vi "Engine Out - HPCR.vi"(4 "Control Inputs":T2={"Engine Speed [RPM]"=0.0, "Engine Status"=enum."STALLED", "Load Control \nMode"=enum."Max Speed Governor", "dt(s)"=0.0, "Number of Cylinders"=0, "Engine Displacement [cc]"=0.0, "StoichAFR"=0.0, "Q.LHV Fuel [kJ/kg]"=0.0, "BattV PSU [V]"=0.0, "12V PSU [V]"=0.0, "5V PSU [V]"=0.0, "Pedal Position [%]"=0.0, "Oil Pressure [kPa]"=0.0, "Oil Temp [C]"=0.0, "Oil Level [%]"=0.0, "Engine Coolant Temp (ECT) [C]"=0.0, "Engine Coolant Pressure [kPa]"=0.0, "Rail Pressure [bar]"=0.0, "Fuel Pressure [kPa]"=0.0, "Fuel Temp [C]"=0.0, "Vacuum Pressure [kPa]"=0.0, "Throttle Position [%]"=0.0, "Cam1 Advance [CAD]"=0.0, "Cam2 Advance [CAD]"=0.0, "Cam3 Advance [CAD]"=0.0, "Cam4 Advance [CAD]"=0.0, "CA50 Control Output [CAD]"=[], "CA50 Control Output Valid"=[], "Intake Air Temp (IAT) [C]"=0.0, "Barometric Air Pressure [kPa]"=0.0, "Intake Air Rel. Humidity [%]"=0.0, "Mass Air Flow (MAF) [kg/hr]"=0.0, "Turbo Inlet Air Pressure [kPa]"=0.0, "Turbo Inlet Air Temp [C]"=0.0, "Turbo Outlet Air Pressure [kPa]"=0.0, "Turbo Outlet Air Temp [C]"=0.0, "CAC Outlet Pressure [kPa]"=0.0, "CAC Outlet Temp [C]"=0.0, "Intake Manifold Pressure (MAP) [kPa]"=0.0, "Intake Manifold Temp (MAT) [C]"=0.0, "Exhaust Manifold Pressure [kPa]"=0.0, "Exhaust Manifold Temp [C]"=0.0, "HighP EGR Cooler Outlet Pressure [kPa]"=0.0, "HighP EGR Cooler Outlet Temp [C]"=0.0, "HighP EGR Differential Pressure [kPa]"=0.0, "HighP EGR Valve Position [%]"=0.0, "Turbo Outlet Exhaust Pressure [kPa]"=0.0, "Turbo Outlet Exhaust Temp [C]"=0.0, "VGT Position 1 [%]"=0.0, "VGT Position 2 [%]"=0.0, "Turbo Speed 1 [RPM]"=0.0, "Turbo Speed 2 [RPM]"=0.0, "LowP EGR Differential Pressure [kPa]"=0.0, "LowP EGR Valve Position [%]"=0.0, "UEGO1Lambda"=0.0, "UEGO1_Hot"=FALSE, "UEGO2Lambda"=0.0, "UEGO2_Hot"=FALSE, "Knock Intensity"=[], "Knock"=[]} {"Knock Intensity" format="%.2f"; "CA50 Control Output [CAD]" format="%.2f"; "Exhaust Manifold Temp [C]" format="%#_6f"; "UEGO2Lambda" format="%.2f"; "Intake Manifold Temp (MAT) [C]" format="%#_6f"; "UEGO1Lambda" format="%.2f"}, 7 "Rail Pressure Setpoint [bar]":sgl format="%.2f") -> (2 "HPV LS Output":T1, 3 "IMV LS Output":T1)   [LabVIEW 2015, in "ECS-RT.lvlib"]
uses:
  ECS-RT.lvlib
  Typedefs/Control Inputs/Control Inputs.ctl
  Typedefs/EPT/Engine Status.ctl
  Typedefs/MISC/Load Control Mode.ctl
  Typedefs/Raw Outputs/LS.ctl
  ECS-Shared.lvlib
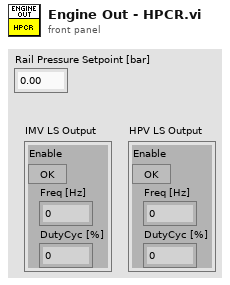
[diagram p1: front panel]
types:
  T1 = typedef "ECS-Shared.lvlib/LS.ctl" = cluster{"Enable":bool, "Freq [Hz]":sgl, "DutyCyc [%]":sgl}
  T2 = typedef "ECS-Shared.lvlib/Control Inputs.ctl" = cluster{"Engine Speed [RPM]":sgl, "Engine Status":T3, "Load Control \nMode":T4, "dt(s)":sgl, "Number of Cylinders":u8, "Engine Displacement [cc]":sgl, "StoichAFR":sgl, "Q.LHV Fuel [kJ/kg]":sgl, "BattV PSU [V]":sgl, "12V PSU [V]":sgl, "5V PSU [V]":sgl, "Pedal Position [%]":sgl, "Oil Pressure [kPa]":sgl, "Oil Temp [C]":sgl, "Oil Level [%]":sgl, "Engine Coolant Temp (ECT) [C]":sgl, "Engine Coolant Pressure [kPa]":sgl, "Rail Pressure [bar]":sgl, "Fuel Pressure [kPa]":sgl, "Fuel Temp [C]":sgl, "Vacuum Pressure [kPa]":sgl, "Throttle Position [%]":sgl, "Cam1 Advance [CAD]":sgl, "Cam2 Advance [CAD]":sgl, "Cam3 Advance [CAD]":sgl, "Cam4 Advance [CAD]":sgl, "CA50 Control Output [CAD]":sgl[], "CA50 Control Output Valid":bool[], "Intake Air Temp (IAT) [C]":sgl, "Barometric Air Pressure [kPa]":sgl, "Intake Air Rel. Humidity [%]":sgl, "Mass Air Flow (MAF) [kg/hr]":sgl, "Turbo Inlet Air Pressure [kPa]":sgl, "Turbo Inlet Air Temp [C]":sgl, "Turbo Outlet Air Pressure [kPa]":sgl, "Turbo Outlet Air Temp [C]":sgl, "CAC Outlet Pressure [kPa]":sgl, "CAC Outlet Temp [C]":sgl, "Intake Manifold Pressure (MAP) [kPa]":sgl, "Intake Manifold Temp (MAT) [C]":sgl, "Exhaust Manifold Pressure [kPa]":sgl, "Exhaust Manifold Temp [C]":sgl, "HighP EGR Cooler Outlet Pressure [kPa]":sgl, "HighP EGR Cooler Outlet Temp [C]":sgl, "HighP EGR Differential Pressure [kPa]":sgl, "HighP EGR Valve Position [%]":sgl, "Turbo Outlet Exhaust Pressure [kPa]":sgl, "Turbo Outlet Exhaust Temp [C]":sgl, "VGT Position 1 [%]":sgl, "VGT Position 2 [%]":sgl, "Turbo Speed 1 [RPM]":sgl, "Turbo Speed 2 [RPM]":sgl, "LowP EGR Differential Pressure [kPa]":sgl, "LowP EGR Valve Position [%]":sgl, "UEGO1Lambda":sgl, "UEGO1_Hot":bool, "UEGO2Lambda":sgl, "UEGO2_Hot":bool, "Knock Intensity":sgl[], "Knock":bool[]}
  T3 = typedef "ECS-Shared.lvlib/Engine Status.ctl" = enum16{"OFF", "STALLED", "CRANKING", "RUNNING", "ACCEL", "DECEL", "SAFE"}
  T4 = typedef "ECS-Shared.lvlib/Load Control Mode.ctl" = enum16{"No Governor", "Min Speed Governor", "Max Speed Governor"}
  T5 = cluster{"PID_Kp":sgl, "PID_Ti":sgl, "PID_Td":sgl, "PID_FF":sgl, "Non-PID_FF":sgl, "PID_Min":sgl, "PID_Max":sgl}
  T6 = cluster{"BattV [V]":sgl, "ValveNominalResitance":sgl, "Min Duty Cycle":sgl, "Manual Max Duty Cycle":sgl, "Manual Duty Cycle":sgl, "Duty Cycle Override":bool, "Drive Frequency":sgl}
  T7 = cluster{"DutyCycle_Output":sgl, "Calculated Max Duty Cycle":sgl, "Valve Current Flow":sgl, "PID_Output":sgl}
  T8 = cluster{"ProportionalAction":sgl, "IntegralAction":sgl, "DerivativeAction":sgl}
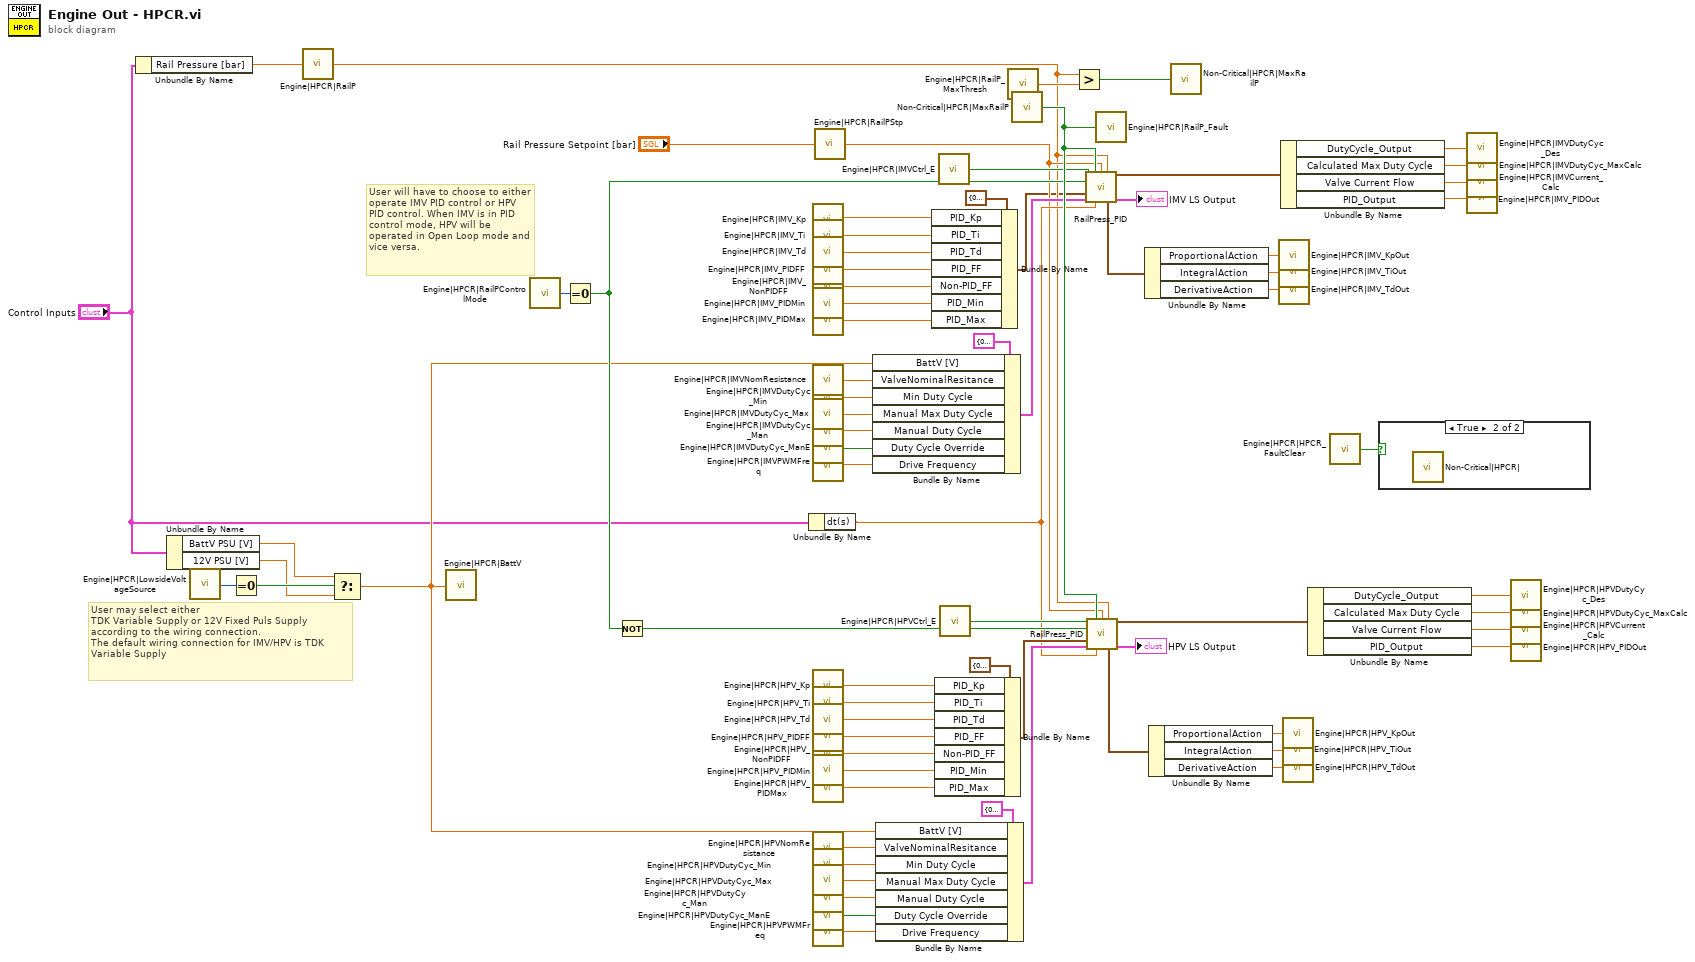
[diagram p0: block diagram]
diagram:
  # "User will have to choose to either operate IMV PID control or HPV PID control. When IMV is in PID control mode, HPV will be operated in Open Loop mode and vice versa."
  # "User may select either\nTDK Variable Supply or 12V Fixed Puls Supply\naccording to the wiring connection.\nThe default wiring connection for IMV/HPV is TDK Variable Supply"
  n1 = Unbundle By Name("Control Inputs") -> ("Rail Pressure [bar]"=w4:sgl)
  n2 = Unbundle By Name("Control Inputs") -> ("BattV PSU [V]"=w11:sgl, "12V PSU [V]"=w10:sgl)
  n3 = call "Engine|HPCR|LowsideVoltageSource"() -> ("Value"=w14:u32)
  n4 = Equal To 0?(x=w14) -> (x = 0?=w13:bool)
  n5 = call "Engine|HPCR|RailP"("Value"=w4) -> ()
  n6 = Select(t=w11, s=w13, f=w10) -> (s? t:f=w12:sgl)
  n7 = call "Engine|HPCR|BattV"("Value"=w12) -> ()
  n8 = call "Engine|HPCR|RailPControlMode"() -> ("Value"=w58:u32)
  n9 = Equal To 0?(x=w58) -> (x = 0?=w59:bool)
  n10 = Not(x=w59) -> (.not. x?=w42:bool)
  n11 = Unbundle By Name("Control Inputs") -> ("dt(s)"=w9:sgl)
  n12 = call "Engine|HPCR|IMV_Kp"() -> ("Value"=w24:sgl)
  n13 = call "Engine|HPCR|IMV_Ti"() -> ("Value"=w25:sgl)
  n14 = call "Engine|HPCR|IMV_Td"() -> ("Value"=w26:sgl)
  n15 = call "Engine|HPCR|IMV_PIDFF"() -> ("Value"=w27:sgl)
  n16 = call "Engine|HPCR|IMV_NonPIDFF"() -> ("Value"=w28:sgl)
  n17 = call "Engine|HPCR|IMV_PIDMin"() -> ("Value"=w29:sgl)
  n18 = call "Engine|HPCR|IMV_PIDMax"() -> ("Value"=w30:sgl)
  n19 = call "Engine|HPCR|IMVNomResistance"() -> ("Value"=w35:sgl)
  n20 = call "Engine|HPCR|IMVDutyCyc_Min"() -> ("Value"=w34:sgl)
  n21 = call "Engine|HPCR|IMVDutyCyc_Max"() -> ("Value"=w36:sgl)
  n22 = call "Engine|HPCR|IMVDutyCyc_Man"() -> ("Value"=w33:sgl)
  n23 = call "Engine|HPCR|IMVDutyCyc_ManE"() -> ("Value"=w32:bool)
  n24 = call "Engine|HPCR|IMVPWMFreq"() -> ("Value"=w31:sgl)
  n25 = call "Engine|HPCR|HPV_Kp"() -> ("Value"=w47:sgl)
  n26 = call "Engine|HPCR|HPV_Ti"() -> ("Value"=w48:sgl)
  n27 = call "Engine|HPCR|HPV_Td"() -> ("Value"=w49:sgl)
  n28 = call "Engine|HPCR|HPV_PIDFF"() -> ("Value"=w50:sgl)
  n29 = call "Engine|HPCR|HPV_NonPIDFF"() -> ("Value"=w51:sgl)
  n30 = call "Engine|HPCR|HPV_PIDMin"() -> ("Value"=w52:sgl)
  n31 = call "Engine|HPCR|HPV_PIDMax"() -> ("Value"=w53:sgl)
  n32 = call "Engine|HPCR|HPVNomResistance"() -> ("Value"=w46:sgl)
  n33 = call "Engine|HPCR|HPVDutyCyc_Min"() -> ("Value"=w54:sgl)
  n34 = call "Engine|HPCR|HPVDutyCyc_Max"() -> ("Value"=w55:sgl)
  n35 = call "Engine|HPCR|HPVDutyCyc_Man"() -> ("Value"=w56:sgl)
  n36 = call "Engine|HPCR|HPVDutyCyc_ManE"() -> ("Value"=w57:bool)
  n37 = call "Engine|HPCR|HPVPWMFreq"() -> ("Value"=w45:sgl)
  n38 = call "Engine|HPCR|RailPStp"("Value"="Rail Pressure Setpoint [bar]") -> ()
  n39 = Bundle By Name(cluster=T6 {"BattV [V]"=0.0, "ValveNominalResitance"=0.0, "Min Duty Cycle"=0.0, "Manual Max Duty Cycle"=0.0, "Manual Duty Cycle"=0.0, "Duty Cycle Override"=FALSE, "Drive Frequency"=0.0} ("Output Management Controls"), "BattV [V]"=w12, "ValveNominalResitance"=w35, "Min Duty Cycle"=w34, "Manual Max Duty Cycle"=w36, "Manual Duty Cycle"=w33, "Duty Cycle Override"=w32, "Drive Frequency"=w31) -> (w23:T6)
  n40 = Bundle By Name(cluster=T6 {"BattV [V]"=0.0, "ValveNominalResitance"=0.0, "Min Duty Cycle"=0.0, "Manual Max Duty Cycle"=0.0, "Manual Duty Cycle"=0.0, "Duty Cycle Override"=FALSE, "Drive Frequency"=0.0} ("Output Management Controls"), "BattV [V]"=w12, "ValveNominalResitance"=w46, "Min Duty Cycle"=w54, "Manual Max Duty Cycle"=w55, "Manual Duty Cycle"=w56, "Duty Cycle Override"=w57, "Drive Frequency"=w45) -> (w44:T6)
  n41 = Bundle By Name(cluster=T5 {"PID_Kp"=0.0, "PID_Ti"=0.01, "PID_Td"=0.0, "PID_FF"=0.0, "Non-PID_FF"=0.0, "PID_Min"=-100.0, "PID_Max"=100.0} ("PID Settings"), "PID_Kp"=w24, "PID_Ti"=w25, "PID_Td"=w26, "PID_FF"=w27, "Non-PID_FF"=w28, "PID_Min"=w29, "PID_Max"=w30) -> (w1:T5)
  n42 = Bundle By Name(cluster=T5 {"PID_Kp"=0.0, "PID_Ti"=0.01, "PID_Td"=0.0, "PID_FF"=0.0, "Non-PID_FF"=0.0, "PID_Min"=-100.0, "PID_Max"=100.0} ("PID Settings"), "PID_Kp"=w47, "PID_Ti"=w48, "PID_Td"=w49, "PID_FF"=w50, "Non-PID_FF"=w51, "PID_Min"=w52, "PID_Max"=w53) -> (w43:T5)
  n43 = call "Engine|HPCR|IMVCtrl_E"() -> ("Value"=w16:bool)
  n44 = call "Engine|HPCR|HPVCtrl_E"() -> ("Value"=w41:bool)
  n45 = call "Engine|HPCR|RailP_MaxThresh"() -> ("Value"=w15:sgl)
  n46 = call "Non-Critical|HPCR|MaxRailP"() -> ("Fault"=w70:bool)  [unwired: 2 in]
  n47 = Greater?(x=w4, y=w15) -> (0:w60:bool)
  n48 = call "RailPress_PID.vi"("Control Enable"=w16, "Fault Input"=w70, "Rail Press Setpoint"="Rail Pressure Setpoint [bar]", "Rail Pressure"=w4, "PID Enable"=w59, "PID Settings"=w1, "Output Management Controls"=w23, "dt (s)"=w9) -> ("Output"=w17:T7, "PID_Action_Output"=w64:T8, "LS Output"=→"IMV LS Output":T1)  [unwired: 5 in]
  n49 = call "RailPress_PID.vi"("Control Enable"=w41, "Fault Input"=w70, "Rail Press Setpoint"="Rail Pressure Setpoint [bar]", "Rail Pressure"=w4, "PID Enable"=w42, "PID Settings"=w43, "Output Management Controls"=w44, "dt (s)"=w9) -> ("Output"=w22:T7, "PID_Action_Output"=w68:T8, "LS Output"=→"HPV LS Output":T1)  [unwired: 5 in]
  n50 = call "Engine|HPCR|RailP_Fault"("Value"=w70) -> ()
  n51 = Unbundle By Name(w64) -> ("ProportionalAction"=w63:sgl, "IntegralAction"=w62:sgl, "DerivativeAction"=w61:sgl)
  n52 = Unbundle By Name(w68) -> ("ProportionalAction"=w65:sgl, "IntegralAction"=w66:sgl, "DerivativeAction"=w67:sgl)
  n53 = call "Non-Critical|HPCR|MaxRailP"("Fault"=w60) -> ()  [unwired: 2 in]
  n54 = call "Engine|HPCR|IMV_KpOut"("Value"=w63) -> ()
  n55 = call "Engine|HPCR|IMV_TiOut"("Value"=w62) -> ()
  n56 = call "Engine|HPCR|IMV_TdOut"("Value"=w61) -> ()
  n57 = Unbundle By Name(w17) -> ("DutyCycle_Output"=w18:sgl, "Calculated Max Duty Cycle"=w19:sgl, "Valve Current Flow"=w20:sgl, "PID_Output"=w21:sgl)
  n58 = call "Engine|HPCR|HPV_KpOut"("Value"=w65) -> ()
  n59 = call "Engine|HPCR|HPV_TiOut"("Value"=w66) -> ()
  n60 = call "Engine|HPCR|HPV_TdOut"("Value"=w67) -> ()
  n61 = Unbundle By Name(w22) -> ("DutyCycle_Output"=w37:sgl, "Calculated Max Duty Cycle"=w38:sgl, "Valve Current Flow"=w39:sgl, "PID_Output"=w40:sgl)
  n62 = call "Engine|HPCR|HPCR_FaultClear"() -> ("Value"=w69:bool)
  n63 = case shown="True" w69 {
    frame False {
    }
    frame True {
      n64 = call "Non-Critical|HPCR|"() -> ()  [unwired: 3 in]
    }
  }
  n65 = call "Engine|HPCR|IMVDutyCyc_Des"("Value"=w18) -> ()
  n66 = call "Engine|HPCR|IMVDutyCyc_MaxCalc"("Value"=w19) -> ()
  n67 = call "Engine|HPCR|IMVCurrent_Calc"("Value"=w20) -> ()
  n68 = call "Engine|HPCR|IMV_PIDOut"("Value"=w21) -> ()
  n69 = call "Engine|HPCR|HPVDutyCyc_Des"("Value"=w37) -> ()
  n70 = call "Engine|HPCR|HPVDutyCyc_MaxCalc"("Value"=w38) -> ()
  n71 = call "Engine|HPCR|HPVCurrent_Calc"("Value"=w39) -> ()
  n72 = call "Engine|HPCR|HPV_PIDOut"("Value"=w40) -> ()
